vi "SOUR_POW_STAR.vi"(0 "VISA IN":refnum<visa-resource-name>, 1 "Start Power":dbl, 5 "error in":errorcluster, 7 "Channel":i32) -> (14 "VISA Out":refnum<visa-resource-name>, 19 "error out":errorcluster)   [LabVIEW 2018, in "PNA-X.lvlib"]
doc: "SOURce<cnum>:POWer:STARt <num> \n(Read-Write) Sets the power sweep start power. Must also set \nSENS:SWE:TYPE POWer and SOURce:POWer:STOP <num>. \nParameters \n<cnum> Any existing channel number. If unspecified, value is set to 1 \n<num> Start power. \nNote: The range of settable power values depends on the PNA model and if \nsource attenuators are installed. To determine the range of values, perform a \nquery using MAX, then MIN, as an argument. (SOUR:POW:ATT:AUTO must \nbe set to ON) Example: SOURce:POWer:STARt? MIN \nActual achievable leveled power depends on frequency. \nExamples SOUR:POW:STAR -15 \nsource2:power:start -7 \nQuery Syntax SOURce<cnum>:POWer:STARt? \nReturn Type Numeric \nDefault 0 dBm"
uses:
  PNA-X.lvlib
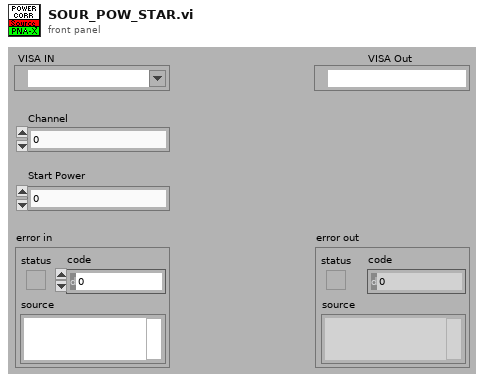
[diagram p1: front panel]
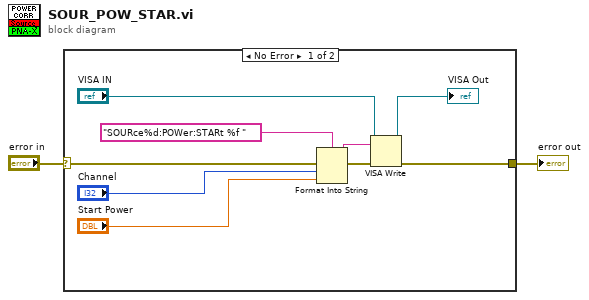
[diagram p0: block diagram]
diagram:
  n1 = case shown="No Error" "error in" {
    selector: "error in" -> [w11 w12]
    tunnel: [w6 w12] -> w1
    frame No Error {
      n2 = Format Into String(format string="SOURce%d:POWer:STARt %f " ("Cmdline"), error in=w11, "Channel", "Start Power") -> (resulting string=w9:string, error out=w10:errorcluster)  [unwired: 1 in]
      n3 = VISA Write(VISA resource name="VISA IN", write buffer=w9, error in (no error)=w10) -> (VISA resource name out=→"VISA Out":refnum<visa-resource-name>, error out=w6:errorcluster)  [unwired: 1 out]
    }
    frame Error {
    }
  }
  "error out" <- w1
